vi "Get Data.vi"(8 "error in (no error)":errorcluster, 11 "CN79000 in":refnum<class "CN79000.lvclass">=refnum) -> (0 "error out":errorcluster, 2 "DataArray":refnum<class "Data.lvclass">[](array[class]), 3 "CN79000 out":refnum<class "CN79000.lvclass">)   [LabVIEW 2014, in "CN79000.lvclass"]
doc: "Retrieve data from the serial device. The data retrieved should be the standard data for the device, but the structure of that data may differ. This is the reason that an array of data class objects is returned rather than a single value."
uses:
  CN79000.lvclass
  Build Command-Single Val.vi
  DataClass/Array Data/Single 1-D/Single_Array.lvclass
  reusable/Data/Array Data/Single 1-D/Single_Array.lvclass
  <vilib>/addons/_NISVFA/_Shared subVIs/Data Objects/Data/Data.lvclass
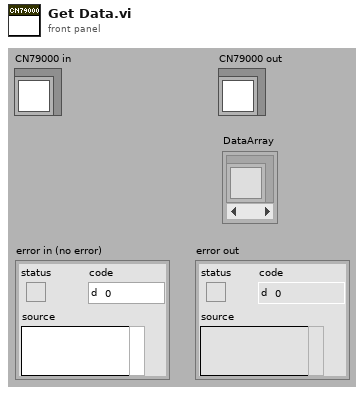
[diagram p1: front panel]
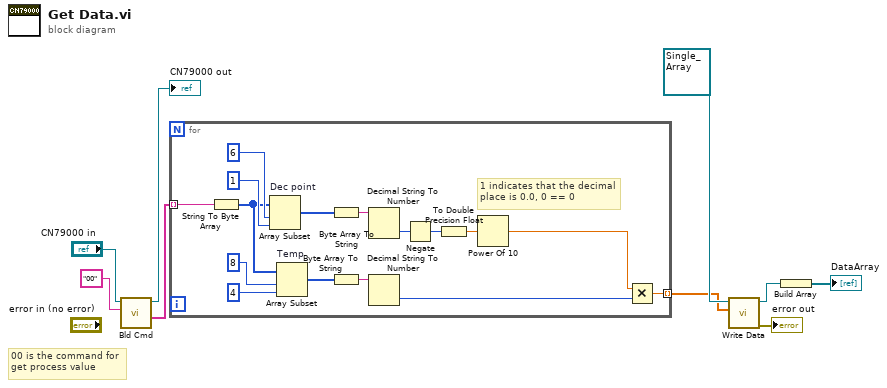
[diagram p0: block diagram]
diagram:
  # "00 is the command for get process value"
  n1 = call-poly "Bld Cmd.vi"("Cmd"="00", "CN79000 in"="CN79000 in") -> ("DataOut"=w7:string[], "CN79000 out"=→"CN79000 out":refnum<class "CN79000.lvclass">)  [unwired: 5 in, 2 out]
  n2 = for {
    tunnel: w7 -> [w11] mode=indexing
    tunnel: [w10] -> w4 mode=indexing
    # "1 indicates that the decimal place is 0.0, 0 == 0"
    n3 = String To Byte Array(string=w11) -> (unsigned byte array=w23:u8[])
    n4 = Array Subset "Dec point"(array=w23, index=6, length=1) -> (w20:u8[])
    n5 = Array Subset "Temp"(array=w23, index=8, length=4) -> (w19:u8[])
    n6 = Byte Array To String(unsigned byte array=w20) -> (string=w18:string)
    n7 = Byte Array To String(unsigned byte array=w19) -> (string=w17:string)
    n8 = Decimal String To Number(string=w18) -> (number=w16:i32)  [unwired: 2 in, 1 out]
    n9 = Decimal String To Number(string=w17) -> (number=w14:i32)  [unwired: 2 in, 1 out]
    n10 = Negate(x=w16) -> (-x=w13:i32)
    n11 = To Double Precision Float(number=w13) -> (double precision float=w12:dbl)
    n12 = Power Of 10(x=w12) -> (10^x=w15:dbl)
    n13 = Multiply(x=w15, y=w14) -> (x*y=w10:dbl)
  }
  n14 = call "Write Data.vi"("Data"=w4, "Single_Array in"=refnum<class "Single_Array.lvclass"> refnum ("Single_Array.lvclass")) -> ("error out"=→"error out":errorcluster, "Single_Array out"=w3:refnum<class "Single_Array.lvclass">)  [unwired: 8 in]
  n15 = Build Array(w3) -> (→"DataArray":refnum<class "Single_Array.lvclass">[])
